vi "Init.vi"(4 "Auto Clear Buffer":bool, 5 "Input Index":i32, 6 "Auto Init Buffer":bool=TRUE, 7 "Output Index":i32, 8 "error in (no error)":errorcluster, 9 "Auto UnLoad":bool, 10 "ONNX Path":path, 11 "ONNX Class in":refnum<class "ONNX Class.lvclass">) -> (0 "error out":errorcluster, 2 "Session ID":i32, 3 "ONNX Class out":refnum<class "ONNX Class.lvclass">)   [LabVIEW 2017, in "ONNX Class Library.lvlib" / "ONNX Class.lvclass"]
uses:
  ONNX Class.lvclass
  ONNX Class Library.lvlib
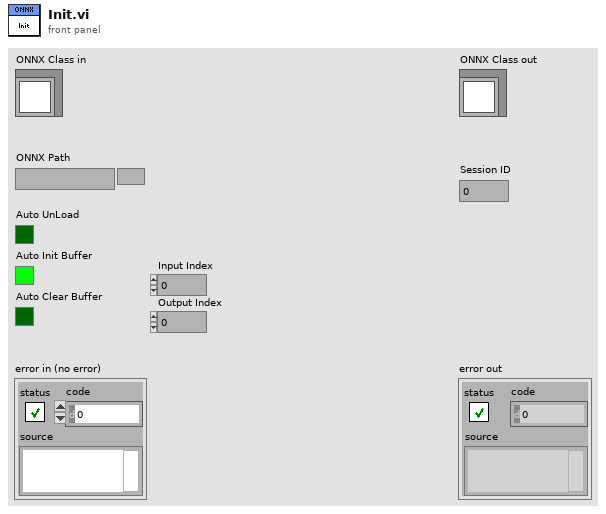
[diagram p1: front panel]
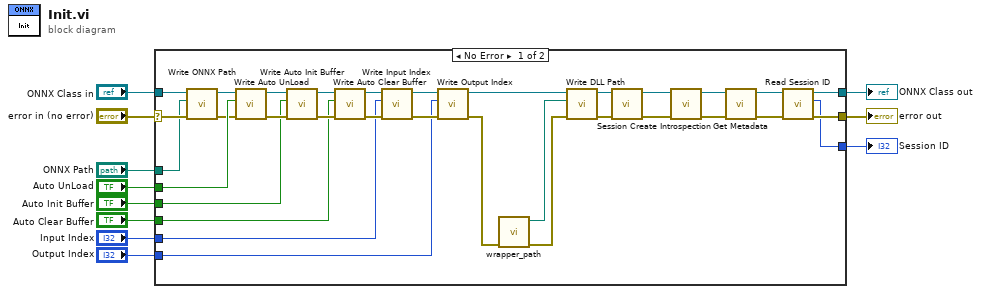
[diagram p0: block diagram]
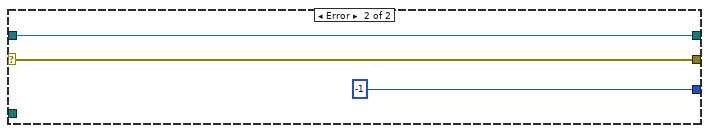
[diagram p2: hidden frame]
diagram:
  n1 = case shown="No Error" "error in (no error)" {
    selector: "error in (no error)" -> [w42 w47]
    tunnel: [w33 w47] -> w10
    tunnel: [w34 w46] -> w8
    tunnel: "ONNX Class in" -> [w44 w46]
    tunnel: "ONNX Path" -> [w41 _]
    tunnel: "Auto UnLoad" -> [w40 _]
    tunnel: [w32 -1 ("Session ID")] -> w5
    tunnel: "Auto Clear Buffer" -> [w27 _]
    tunnel: "Auto Init Buffer" -> [w26 _]
    tunnel: "Output Index" -> [w19 _]
    tunnel: "Input Index" -> [w18 _]
    frame No Error {
      n2 = call-dynamic "Write ONNX Path.vi"("error in (no error)"=w42, "ONNX Path"=w41, "ONNX Class in"=w44) -> ("error out"=w39:errorcluster, "ONNX Class out"=w43:refnum<class "ONNX Class.lvclass">)  [unwired: 7 in]
      n3 = call-dynamic "Write Auto UnLoad.vi"("error in (no error)"=w39, "Auto UnLoad"=w40, "ONNX Class in"=w43) -> ("error out"=w29:errorcluster, "ONNX Class out"=w31:refnum<class "ONNX Class.lvclass">)  [unwired: 7 in]
      n4 = call-dynamic "Write Auto Init Buffer.vi"("error in (no error)"=w29, "Auto Init Buffer"=w26, "ONNX Class in"=w31) -> ("error out"=w28:errorcluster, "ONNX Class out"=w30:refnum<class "ONNX Class.lvclass">)  [unwired: 7 in]
      n5 = call-dynamic "Write Auto Clear Buffer.vi"("error in (no error)"=w28, "Auto Clear Buffer"=w27, "ONNX Class in"=w30) -> ("error out"=w25:errorcluster, "ONNX Class out"=w24:refnum<class "ONNX Class.lvclass">)  [unwired: 7 in]
      n6 = call-dynamic "Write Input Index.vi"("error in (no error)"=w25, "Input Index"=w18, "ONNX Class in"=w24) -> ("error out"=w22:errorcluster, "ONNX Class out"=w23:refnum<class "ONNX Class.lvclass">)  [unwired: 7 in]
      n7 = call-dynamic "Write Output Index.vi"("error in (no error)"=w22, "Output Index"=w19, "ONNX Class in"=w23) -> ("error out"=w20:errorcluster, "ONNX Class out"=w21:refnum<class "ONNX Class.lvclass">)  [unwired: 7 in]
      n8 = call "wrapper_path.vi"("error in (no error)"=w20) -> ("error out"=w37:errorcluster, "wrapper path"=w38:path)  [unwired: 9 in]
      n9 = call-dynamic "Write DLL Path.vi"("error in (no error)"=w37, "DLL Path"=w38, "ONNX Class in"=w21) -> ("error out"=w35:errorcluster, "ONNX Class out"=w36:refnum<class "ONNX Class.lvclass">)  [unwired: 7 in]
      n10 = call-dynamic "Session Create.vi"("error in (no error)"=w35, "ONNX Class in"=w36) -> ("error out"=w16:errorcluster, "ONNX Class out"=w17:refnum<class "ONNX Class.lvclass">)  [unwired: 8 in]
      n11 = call-dynamic "Introspection.vi"("error in (no error)"=w16, "ONNX Class in"=w17) -> ("error out"=w14:errorcluster, "ONNX Class out"=w15:refnum<class "ONNX Class.lvclass">)  [unwired: 6 in, 2 out]
      n12 = call-dynamic "Get Metadata.vi"("error in (no error)"=w14, "ONNX Class in"=w15) -> ("error out"=w12:errorcluster, "ONNX Class out"=w13:refnum<class "ONNX Class.lvclass">)  [unwired: 7 in, 1 out]
      n13 = call-dynamic "Read Session ID.vi"("error in (no error)"=w12, "ONNX Class in"=w13) -> ("error out"=w33:errorcluster, "Session ID"=w32:i32, "ONNX Class out"=w34:refnum<class "ONNX Class.lvclass">)  [unwired: 7 in]
    }
    frame Error {
    }
  }
  "error out" <- w10
  "ONNX Class out" <- w8
  "Session ID" <- w5
